vi "Get All Occupancy Grid Cells.vi"(8 "error in (no error)":errorcluster, 11 "map reference in":refnum<data-value>) -> (0 "error out":errorcluster, 2 "occupancy grid":dbl[][](array[numeric]), 3 "map reference out":refnum<data-value>)   [LabVIEW 2017, in "NI_Robotics_OccupancyGridWorldMap.lvclass"]
doc: "Returns an array of the cells in an occupancy grid map."
uses:
  <vilib>/robotics/Navigation/shared/WorldMap/OccupancyGridWorldMap/NI_Robotics_OccupancyGridWorldMap.lvclass
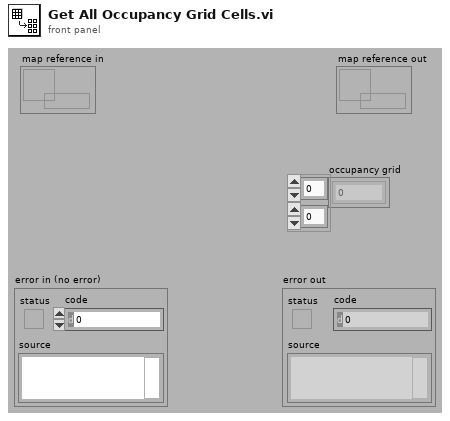
[diagram p1: front panel]
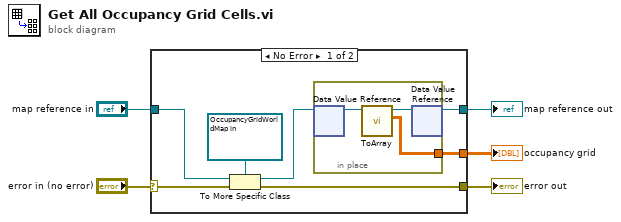
[diagram p0: block diagram]
diagram:
  n1 = case shown="No Error" "error in (no error)" {
    selector: "error in (no error)" -> [w10 w17]
    tunnel: [w12 w16] -> w5
    tunnel: [w11 _] -> w4
    tunnel: [w6 w17] -> w3
    tunnel: "map reference in" -> [w9 w16]
    frame No Error {
      n2 = To More Specific Class(target class=refnum<data-value> refnum ("World Map Reference"), reference=w9, error in=w10) -> (specific class reference=w8:refnum<data-value>, error out=w6:errorcluster)
      n3 = in-place {
        in-place-border: [w13] -> w11
        n4 = in-place-dvr #1(w8) -> (w15:refnum<class "NI_Robotics_OccupancyGridWorldMap.lvclass">)  [unwired: 1 out]
        n5 = call <vilib>:"ToArray.vi"("OccupancyGridWorldMap in"=w15) -> ("cost array"=w13:dbl[][], "OccupancyGridWorldMap out"=w14:refnum<class "NI_Robotics_OccupancyGridWorldMap.lvclass">)  [unwired: 9 in]
        n6 = in-place-dvr #1(w14) -> (w12:refnum<data-value>)  [unwired: 1 out]
      }
    }
    frame Error {
    }
  }
  "error out" <- w3
  "map reference out" <- w5
  "occupancy grid" <- w4
